vi "PS_test.vi"() -> ()   [LabVIEW 2020]
uses:
  IT-M3400.lvlib
panel:
  in  "Battery Type":T1(ring)
  in  "Charge/discharge":enum8{"Charge", "Discharge"}(ring)
  in  "PS error in":errorcluster caption="PS error in (no error)"
  in  "PS VISA in":refnum<visa-resource-name>
  in  "Current Setpoint":dbl format="%#.6g"
  in  "Current Cutoff":dbl
  in  "Charge/Discharge Voltage Setpoint":dbl format="%#.6g"
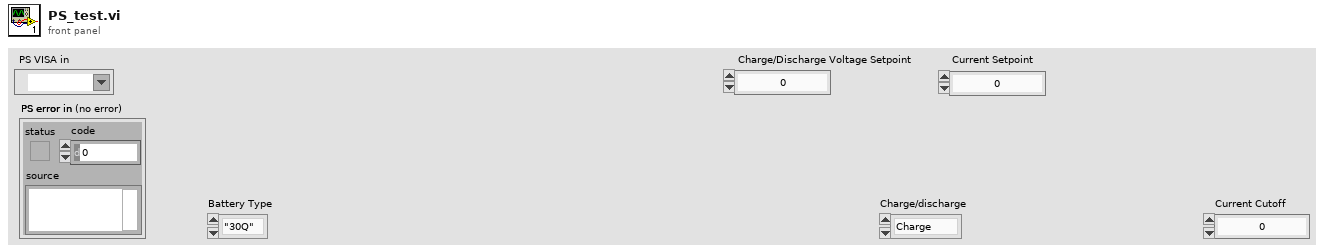
[diagram p1: front panel]
types:
  T1 = enum16{"\"30Q\"", "\"40T\"", "\"2P30Q\"", "\"3P30Q\"", "\"Nissan Leaf\""}
  T2 = cluster{"Baud Rate":u32, "Parity":u16, "Data Bits":u16, "Stop Bits":u16, "Flow Control":u16}
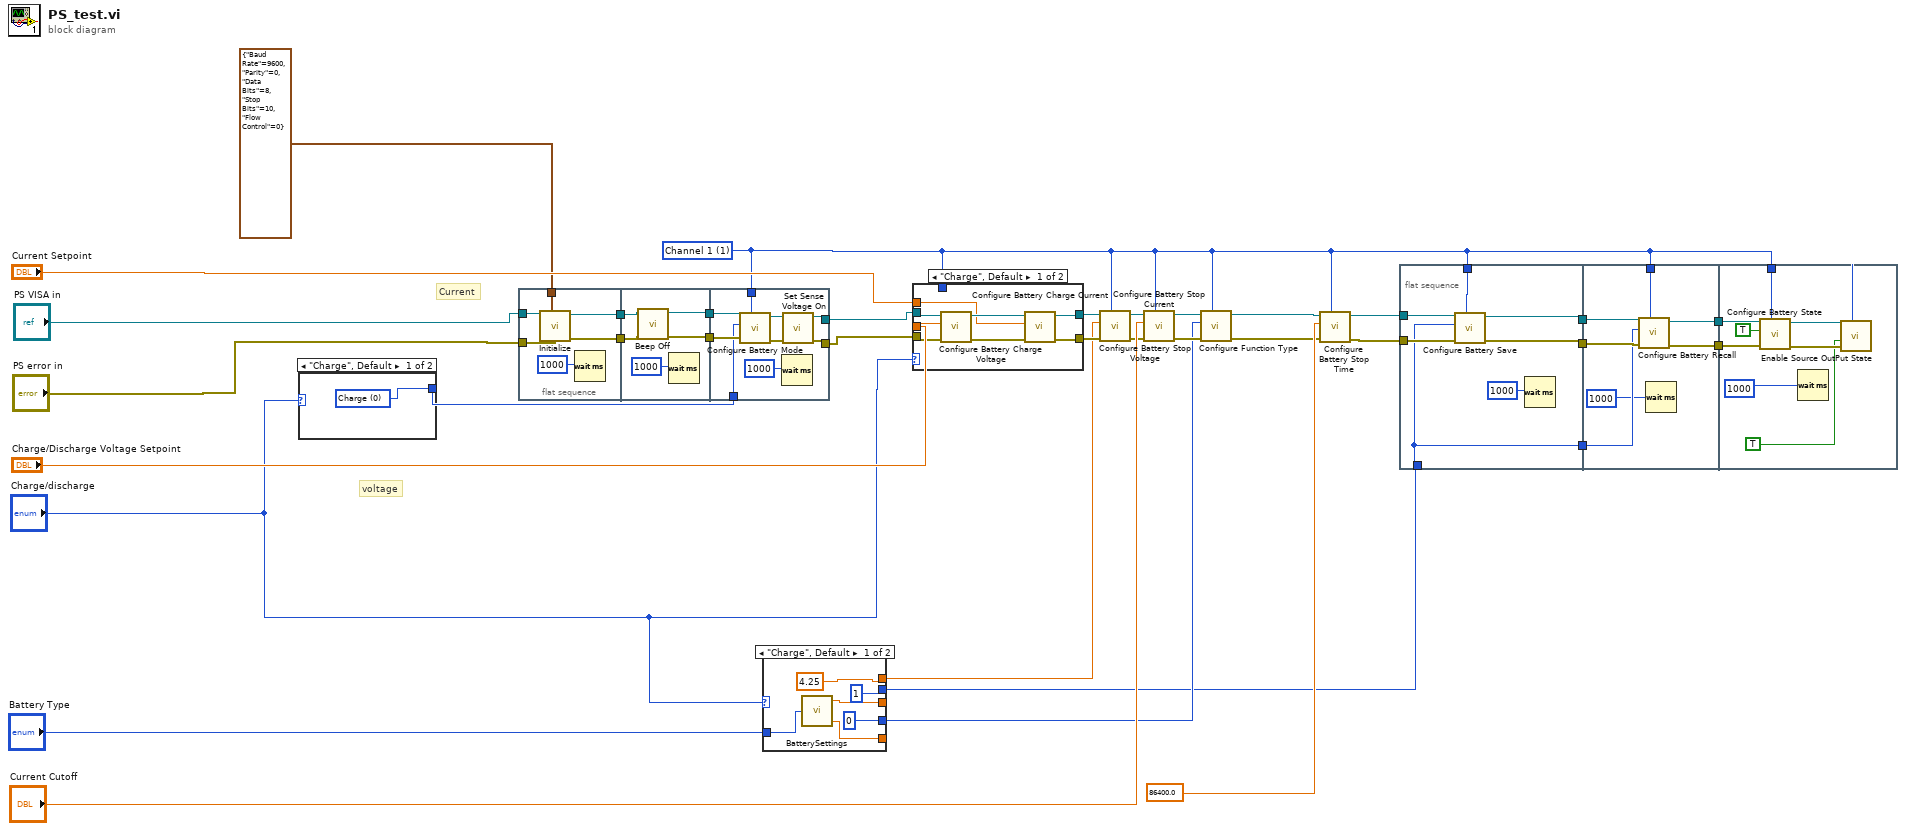
[diagram p0: block diagram]
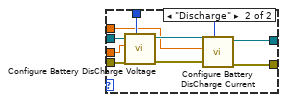
[diagram p2: hidden frame]
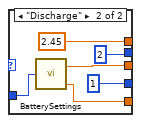
[diagram p3: hidden frame]
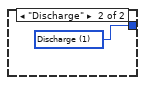
[diagram p4: hidden frame]
diagram:
  w5 = 1 items=["Channel 1"=1, "Channel 2"=2, "Channel 3"=3, "Channel 4"=4, "Channel 5"=5, "Channel 6"=6, "Channel 7"=7, "Channel 8"=8, "Channel 8"=9, "Channel 10"=10, "Channel 11"=11, "Channel 12"=12, "Channel 13"=13, "Channel 14"=14, "Channel 15"=15, "Channel 16"=16] ("Channel")
  # "voltage"
  # "Current"
  n1 = case shown="\"Charge\", Default" "Charge/discharge" {
    tunnel: [w36 w37] -> w8
    frame "Charge", Default {
      w36 = u8 0 items=["Charge", "Discharge"] ("Battery Mode")
    }
    frame "Discharge" {
      w37 = u8 1 items=["Charge", "Discharge"] ("Battery Mode")
    }
  }
  n2 = flat-sequence {
    tunnel: T2 {"Baud Rate"=9600, "Parity"=0, "Data Bits"=8, "Stop Bits"=10, "Flow Control"=0} ("Serial Configuration") -> [w43]
    tunnel: "PS error in" -> [w42]
    tunnel: "PS VISA in" -> [w41]
    tunnel: [w39] -> w30
    tunnel: [w38] -> w29
    tunnel: [w47] -> w28
    tunnel: [w46] -> w27
    tunnel: w30 -> [w45]
    tunnel: w29 -> [w44]
    tunnel: w28 -> [w55]
    tunnel: w27 -> [w56]
    tunnel: w5 -> [w57]
    tunnel: [w50] -> w3
    tunnel: [w51] -> w4
    tunnel: w8 -> [w49]
    frame #0 {
      n3 = call "Initialize.vi"("Serial Configuration"=w43, "error in"=w42, "VISA resource name"=w41) -> ("error out"=w38:errorcluster, "VISA resource name out"=w39:refnum<visa-resource-name>)  [unwired: 7 in]
      n4 = Wait (ms)(milliseconds to wait=1000) -> ()  [unwired: 1 out]
    }
    frame #1 {
      n5 = call "Beep Off.vi"("error in"=w44, "VISA resource name"=w45) -> ("error out"=w46:errorcluster, "VISA resource name out"=w47:refnum<visa-resource-name>)  [unwired: 8 in]
      n6 = Wait (ms)(milliseconds to wait=1000) -> ()  [unwired: 1 out]
    }
    frame #2 {
      n7 = call "Configure Battery Mode.vi"("Channel"=w57, "error in"=w56, "Battery Mode"=w49, "VISA resource name"=w55) -> ("error out"=w52:errorcluster, "VISA resource name out"=w53:refnum<visa-resource-name>)  [unwired: 6 in]
      n8 = Wait (ms)(milliseconds to wait=1000) -> ()  [unwired: 1 out]
      n9 = call "Set Sense Voltage On.vi"("error in"=w52, "VISA resource name"=w53) -> ("error out"=w50:errorcluster, "VISA resource name out"=w51:refnum<visa-resource-name>)  [unwired: 8 in]
    }
  }
  n10 = case shown="\"Charge\", Default" "Charge/discharge" {
    tunnel: "Battery Type" -> [w63 w69]
    tunnel: [w62 w67] -> _
    tunnel: [u8 0 ("File") u8 1 ("File")] -> w12
    tunnel: [u8 1 ("File") u8 2 ("File")] -> w11
    tunnel: [w59 w65] -> _
    tunnel: [4.25 2.45] -> w10
    frame "Charge", Default {
      n11 = call "BatterySettings.vi"("Battery Type"=w63) -> ("RatedCapacity (Ah)"=w59:dbl, "Max Voltage (V)"=w62:dbl)  [unwired: 2 in, 1 out]
    }
    frame "Discharge" {
      n12 = call "BatterySettings.vi"("Battery Type"=w69) -> ("RatedCapacity (Ah)"=w65:dbl, "Min Voltage (V)"=w67:dbl)  [unwired: 2 in, 1 out]
    }
  }
  n13 = case shown="\"Charge\", Default" "Charge/discharge" {
    tunnel: w4 -> [w77 w86]
    tunnel: w3 -> [w76 w85]
    tunnel: [w71 w82] -> w19
    tunnel: [w70 w81] -> w18
    tunnel: w5 -> [_ w80]
    tunnel: "Charge/Discharge Voltage Setpoint" -> [w73 w79]
    tunnel: "Current Setpoint" -> [w72 w78]
    frame "Charge", Default {
      n14 = call "Configure Battery Charge Voltage.vi"("error in"=w76, "Charge Voltage(V)"=w73, "VISA resource name"=w77) -> ("error out"=w74:errorcluster, "VISA resource name out"=w75:refnum<visa-resource-name>)  [unwired: 6 in]
      n15 = call "Configure Battery Charge Current.vi"("error in"=w74, "Charge Current(A)"=w72, "VISA resource name"=w75) -> ("error out"=w70:errorcluster, "VISA resource name out"=w71:refnum<visa-resource-name>)  [unwired: 7 in]
    }
    frame "Discharge" {
      n16 = call "Configure Battery DisCharge Voltage.vi"("Channel"=w80, "error in"=w85, "Discharge Voltage(V)"=w79, "VISA resource name"=w86) -> ("error out"=w83:errorcluster, "VISA resource name out"=w84:refnum<visa-resource-name>)  [unwired: 6 in]
      n17 = call "Configure Battery DisCharge Current.vi"("Channel"=w80, "error in"=w83, "Discharge Current(A)"=w78, "VISA resource name"=w84) -> ("error out"=w81:errorcluster, "VISA resource name out"=w82:refnum<visa-resource-name>)  [unwired: 6 in]
    }
  }
  n18 = call "Configure Battery Stop Voltage.vi"("Channel"=w5, "error in"=w18, "Stop Voltage(V)"=w10, "VISA resource name"=w19) -> ("error out"=w20:errorcluster, "VISA resource name out"=w21:refnum<visa-resource-name>)  [unwired: 6 in]
  n19 = call "Configure Battery Stop Current.vi"("Channel"=w5, "error in"=w20, "Stop Current(A)"="Current Cutoff", "VISA resource name"=w21) -> ("error out"=w13:errorcluster, "VISA resource name out"=w14:refnum<visa-resource-name>)  [unwired: 6 in]
  n20 = call "Configure Function Type.vi"("Channel"=w5, "error in"=w13, "Function Type"=w12, "VISA resource name"=w14) -> ("error out"=w1:errorcluster, "VISA resource name out"=w2:refnum<visa-resource-name>)  [unwired: 6 in]
  n21 = call "Configure Battery Stop Time.vi"("Channel"=w5, "error in"=w1, "Stop Time(S)"=86400.0, "VISA resource name"=w2) -> ("error out"=w16:errorcluster, "VISA resource name out"=w15:refnum<visa-resource-name>)  [unwired: 6 in]
  n22 = flat-sequence {
    tunnel: w11 -> [w92]
    tunnel: w5 -> [w87]
    tunnel: [w90] -> w35
    tunnel: [w92] -> w34
    tunnel: [w89] -> w33
    tunnel: w16 -> [w93]
    tunnel: w15 -> [w91]
    tunnel: [w96] -> w32
    tunnel: [w97] -> w31
    tunnel: w35 -> [w100]
    tunnel: w34 -> [w99]
    tunnel: w33 -> [w98]
    tunnel: w5 -> [w94]
    tunnel: w5 -> [w102]
    tunnel: w32 -> [w108]
    tunnel: w31 -> [w107]
    frame #0 {
      n23 = call "Configure Battery Save.vi"("Channel"=w87, "error in"=w93, "File"=w92, "VISA resource name"=w91) -> ("error out"=w90:errorcluster, "VISA resource name out"=w89:refnum<visa-resource-name>)  [unwired: 6 in]
      n24 = Wait (ms)(milliseconds to wait=1000) -> ()  [unwired: 1 out]
    }
    frame #1 {
      n25 = call "Configure Battery Recall.vi"("Channel"=w94, "error in"=w100, "File"=w99, "VISA resource name"=w98) -> ("error out"=w97:errorcluster, "VISA resource name out"=w96:refnum<visa-resource-name>)  [unwired: 6 in]
      n26 = Wait (ms)(milliseconds to wait=1000) -> ()  [unwired: 1 out]
    }
    frame #2 {
      n27 = call "Configure Battery State.vi"("Channel"=w102, "error in"=w107, "State"=TRUE, "VISA resource name"=w108) -> ("error out"=w105:errorcluster, "VISA resource name out"=w106:refnum<visa-resource-name>)  [unwired: 6 in]
      n28 = Wait (ms)(milliseconds to wait=1000) -> ()  [unwired: 1 out]
      n29 = call "Enable Source OutPut State.vi"("Channel"=w102, "error in"=w105, "State"=TRUE ("Enable Output|Intput"), "VISA resource name"=w106) -> ()  [unwired: 6 in, 2 out]
    }
  }
